vi "Read Enabled Test Methods.vi"(11 "LUnit Test Case In":refnum<class "LUnit Test Case.lvclass">) -> (1 "Paths":path[](array[path]), 2 "Names":string[](array[string]), 3 "LUnit Test Case Out":refnum<class "LUnit Test Case.lvclass">)   [LabVIEW 2020, in "LUnit Test Case.lvclass"]
uses:
  LUnit Test Case.lvclass
  LUnit Test Case.lvclass/LUnit Test Case.ctl
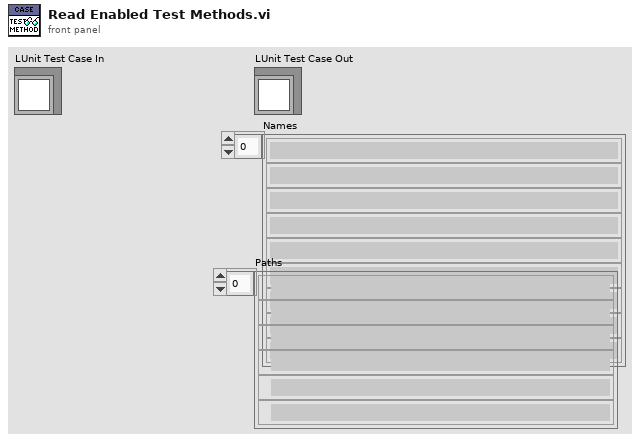
[diagram p1: front panel]
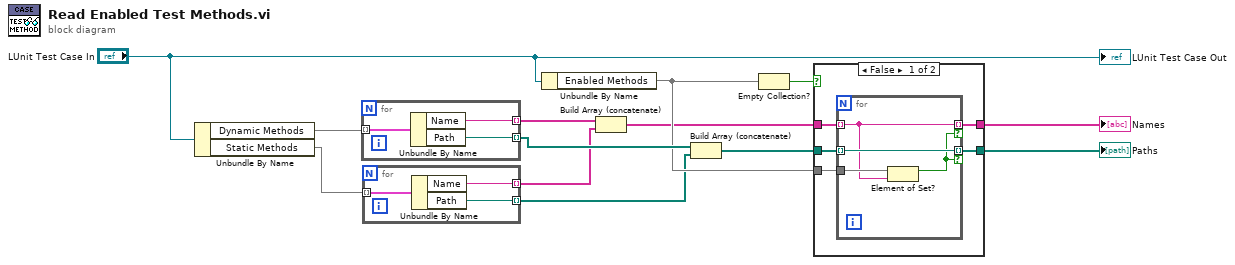
[diagram p0: block diagram]
diagram:
  n1 = Unbundle By Name("LUnit Test Case In") -> ("Dynamic Methods"=w6:map{string, path}, "Static Methods"=w4:map{string, path})
  n2 = for {
    tunnel: w6 -> [w16] mode=indexing
    tunnel: [w14] -> w11 mode=indexing
    tunnel: [w15] -> w10 mode=indexing
    n3 = Unbundle By Name(w16) -> ("Name"=w15:string, "Path"=w14:path)
  }
  n4 = for {
    tunnel: w4 -> [w19] mode=indexing
    tunnel: [w17] -> w1 mode=indexing
    tunnel: [w18] -> w2 mode=indexing
    n5 = Unbundle By Name(w19) -> ("Name"=w18:string, "Path"=w17:path)
  }
  n6 = Unbundle By Name("LUnit Test Case In") -> ("Enabled Methods"=w9:set{string})
  n7 = Build Array (concatenate)(w10, w2) -> (w5:string[])
  n8 = Build Array (concatenate)(w11, w1) -> (w3:path[])
  n9 = Empty Collection?(1:w9) -> (0:w8:bool)
  n10 = case shown="False" w8 {
    tunnel: [w22 w30] -> w12
    tunnel: w3 -> [w21 w30]
    tunnel: w9 -> [w24 _]
    tunnel: w5 -> [w23 w29]
    tunnel: [w20 w29] -> w13
    frame False {
      n11 = for {
        tunnel: w24 -> [w28]
        tunnel: w23 -> [w26] mode=indexing
        tunnel: [w27] -> w22 mode=indexing if=w25
        tunnel: w21 -> [w27] mode=indexing
        tunnel: [w26] -> w20 mode=indexing if=w25
        n12 = Element of Set?(10:w26, 11:w28) -> (3:w25:bool)
      }
    }
    frame True {
    }
  }
  "Names" <- w13
  "Paths" <- w12
  "LUnit Test Case Out" <- "LUnit Test Case In"
